vi "slscswitch Can Connect Channels.vi"(8 "error in (no error)":errorcluster, 9 "channel 2":string, 10 "channel 1":string, 11 "SLSC Switch in":refnum<class "SLSC Switch.lvclass">) -> (0 "error out":errorcluster, 2 "path capability":T1=1 items=["Path Available"=1, "Path Exists"=2, "Path Unsupported"=3, "Resource in Use"=4, "Source Conflict"=5, "Channel Not Available"=6], 3 "SLSC Switch out":refnum<class "SLSC Switch.lvclass">)   [LabVIEW 2015, in "SLSC Switch.lvclass"]
uses:
  SLSC Switch.lvclass
  Path Capability.ctl
  SLSC Switch.lvclass/SLSC Switch.ctl
  Route Manager/Route Manager.lvclass
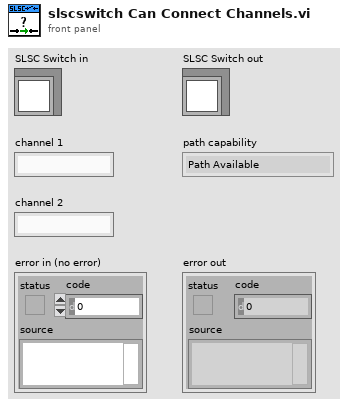
[diagram p1: front panel]
types:
  T1 = typedef "SLSC Switch.lvclass/Path Capability.ctl" = i32
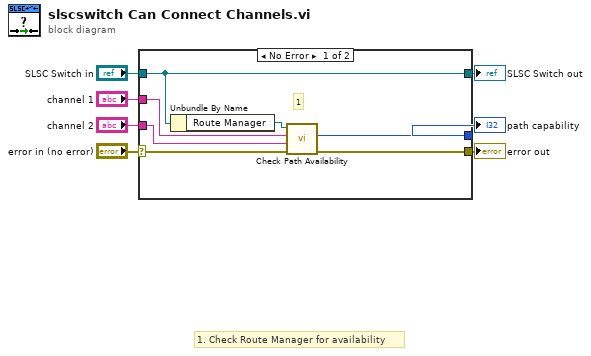
[diagram p0: block diagram]
diagram:
  # "1. Check Route Manager for availability"
  n1 = case shown="No Error" "error in (no error)" {
    selector: "error in (no error)" -> [w14 w16]
    tunnel: [w13 w16] -> w6
    tunnel: [w9 w15] -> w4
    tunnel: "SLSC Switch in" -> [w9 w15]
    tunnel: "channel 1" -> [w12 _]
    tunnel: "channel 2" -> [w11 _]
    tunnel: [w10 _] -> w1
    frame No Error {
      # "1"
      n2 = Unbundle By Name(w9) -> ("Route Manager"=w8:refnum<class "Route Manager.lvclass">)
      n3 = call "Check Path Availability.vi"("error in (no error)"=w14, "channel 2"=w11, "channel 1"=w12, "Route Manager in"=w8) -> ("error out"=w13:errorcluster, "path capability"=w10:T1)  [unwired: 6 in]
    }
    frame Error {
    }
  }
  "error out" <- w6
  "SLSC Switch out" <- w4
  "path capability" <- w1
